vi "Fire Detector.vi"(1 "C02 Level Input":dbl(knob) min=0.0 max=20.0 step=1.0 scale=0.0..20.0) -> (0 "Boolean":bool)   [LabVIEW 2019]
panel:
  out "Average CO2":dbl
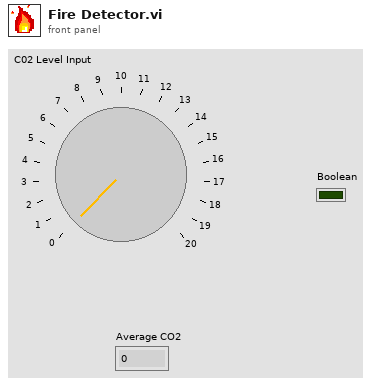
[diagram p1: front panel]
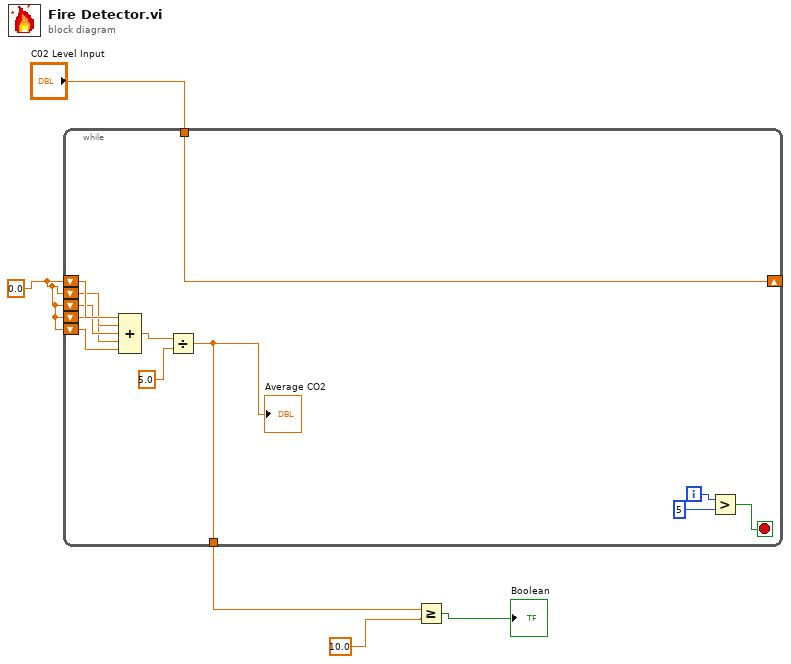
[diagram p0: block diagram]
diagram:
  w5 = 0.0
  n1 = while {
    shift-right: [w7] -> _
    shift-left: w5 -> [w10]
    shift-left: w5 -> [w11]
    shift-left: w5 -> [w12]
    shift-left: w5 -> [w13]
    shift-left: w5 -> [w14]
    tunnel: "C02 Level Input" -> [w7]
    tunnel: [w6] -> w3
    i -> [w17]
    stop <- w16 stop-if-true
    n2 = Compound Arithmetic op=ADD(w14, w13, w12, w11, w10) -> (w9:dbl)
    n3 = Divide(x=w9, y=5.0) -> (x/y=w6:dbl)
    "Average CO2" <- w6
    n4 = Greater?(x=w17, y=5) -> (0:w16:bool)
  }
  n5 = Greater Or Equal?(x=w3, y=10.0) -> (x >= y?=→"Boolean":bool)
